vi "MTM2_logEvent_forceBalanceSystemStatus.vi"(8 "error in (no error)":errorcluster, 11 "logevent_forceBalanceSystemStatus_Ctl":T1) -> (0 "error out":errorcluster, 2 "function return":i32, 3 "logevent_forceBalanceSystemStatus_Ctl out":T1)   [LabVIEW 2018, in "SALLV_MTM2.lvlib"]
doc: "int MTM2_shm_logEvent_forceBalanceSystemStatusLV(MTM2_logevent_forceBalanceSystemStatusLV *logevent_forceBalanceSystemStatus_Ctl );"
uses:
  DataTypes/logevent_forceBalanceSystemStatus.ctl
  SALLV_MTM2.lvlib
  SALLV_MTM2.so
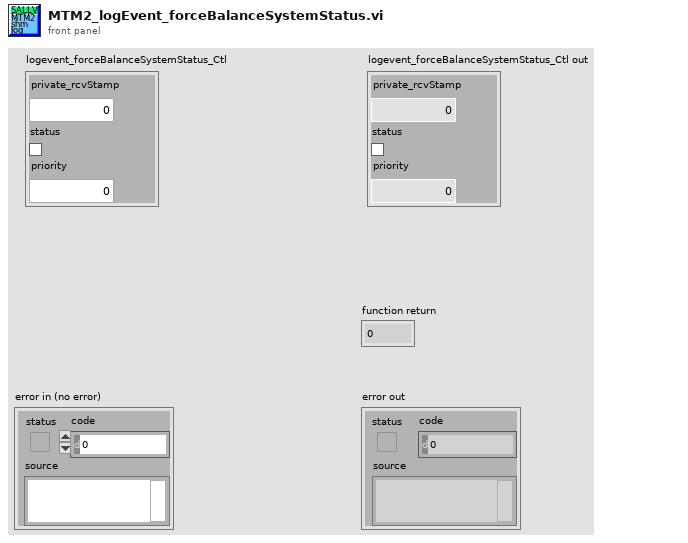
[diagram p1: front panel]
types:
  T1 = typedef "SALLV_MTM2.lvlib/logevent_forceBalanceSystemStatus.ctl" = cluster{"private_rcvStamp":dbl, "status":bool, "priority":i32}
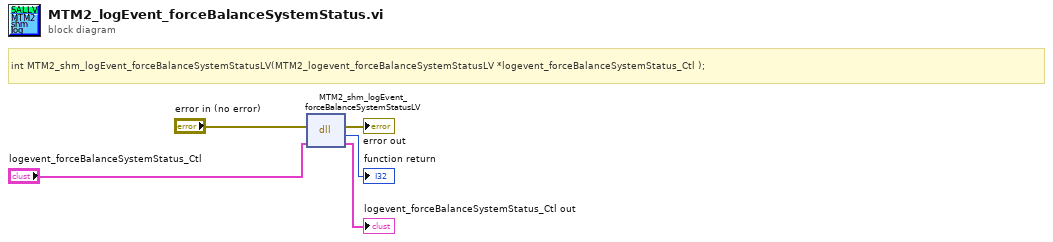
[diagram p0: block diagram]
diagram:
  # "int MTM2_shm_logEvent_forceBalanceSystemStatusLV(MTM2_logevent_forceBalanceSystemStatusLV *logevent_forceBalanceSystemStatus_Ctl );"
  n1 = dll-call lib="home/ttsai/Documents/salTestLabViewApi/SALLV_MTM2/SALLV_MTM2.*" fn="MTM2_shm_logEvent_forceBalanceSystemStatusLV"(error in="error in (no error)", "logevent_forceBalanceSystemStatus_Ctl"="logevent_forceBalanceSystemStatus_Ctl") -> (error out=→"error out":errorcluster, →"function return":i32, "logevent_forceBalanceSystemStatus_Ctl"=→"logevent_forceBalanceSystemStatus_Ctl out":T1)  [unwired: 2 in, 1 out]
